vi "setUp.vi"(8 "error in (no error)":errorcluster, 11 "reference in":refnum<class "RT Start.lvclass">) -> (0 "error out":errorcluster, 3 "reference out":refnum<class "RT Start.lvclass">)   [LabVIEW 2016, in "RT Start.lvclass"]
doc: "setUp runs prior to the test method during test execution. Use this method to initialize any object data required by your tests."
uses:
  RT Start.lvclass
  D:/Programs/National Instruments/LabVIEW 2016/vi.lib/addons/_JKI Toolkits/VI Tester/TestCase.llb/TestCase.lvclass
  <vilib>/addons/_JKI Toolkits/VI Tester/TestCase.llb/TestCase.lvclass
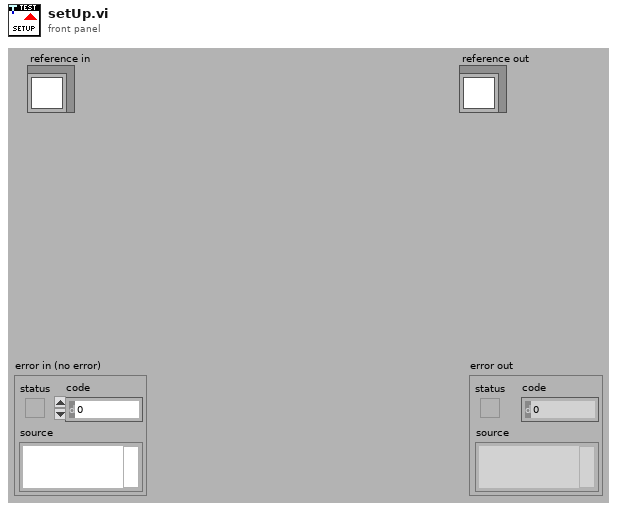
[diagram p1: front panel]
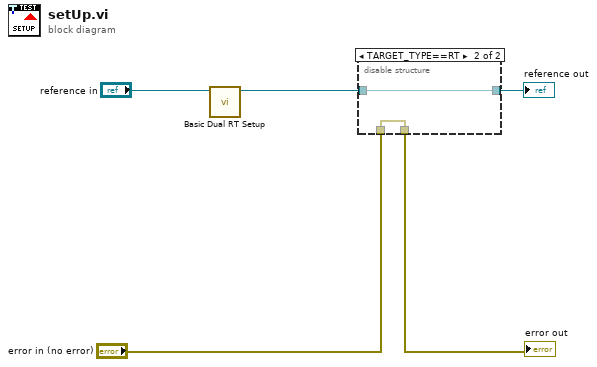
[diagram p0: block diagram]
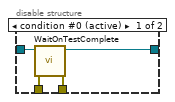
[diagram p2: hidden frame]
diagram:
  n1 = call-dynamic "Basic Dual RT Setup.vi"("1553 Test in"="reference in") -> ("1553 Test out"=w1:refnum<class "RT Start.lvclass">)  [unwired: 9 in, 1 out]
  n2 = disable-structure shown="TARGET_TYPE==RT" {
    disable-tunnel: "error in (no error)" -> [w9 w10]
    disable-tunnel: [w8 w10] -> w4
    disable-tunnel: [w7 w11] -> w3
    disable-tunnel: w1 -> [w6 w11]
    frame condition #0 (active) {
      n3 = call <vilib>:"WaitOnTestComplete.vi"("error in (no error)"=w9, "TestCase in"=w6) -> ("error out"=w8:errorcluster, "TestCase out"=w7:refnum<class "RT Start.lvclass">)  [unwired: 8 in]
    }
    frame condition #1 {
    }
  }
  "error out" <- w4
  "reference out" <- w3
